vi "Charact Result Collection.vi"(0 "Operation":T1, 5 "Index":i32=1, 7 "Path cal resut In":variant) -> (4 "Path cal result out":variant, 6 "All path cal results":variant[](array[variant]))   [LabVIEW 2023, in "RFFixtureCharact.Public.lvlib"]
uses:
  RFFixtureCharact.Public.lvlib
  Type Definitions/Collection Operation.ctl
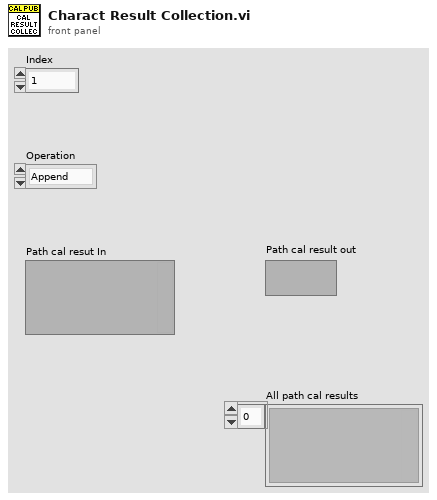
[diagram p1: front panel]
types:
  T1 = typedef "RFFixtureCharact.Public.lvlib/Collection Operation.ctl" = enum16{"Append", "Get", "Get All", "Clear"}
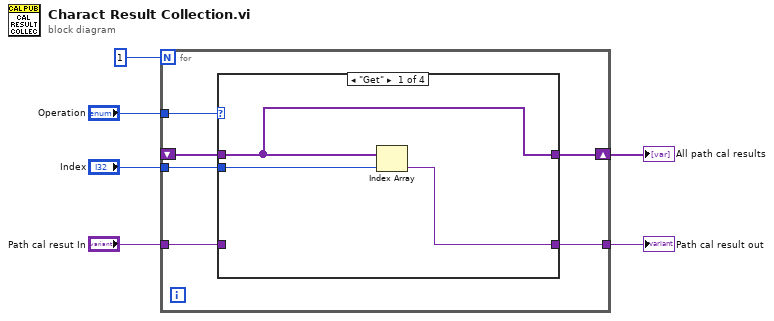
[diagram p0: block diagram]
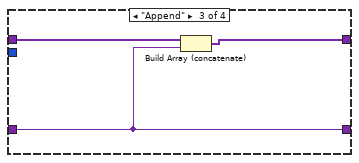
[diagram p3: hidden frame]
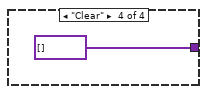
[diagram p4: hidden frame]
diagram:
  n1 = for {
    N: 1 -> [_]
    tunnel: [w12] -> w5
    shift-right: [w9] -> w1
    shift-left: _ -> [w10]
    tunnel: "Path cal resut In" -> [w11]
    tunnel: "Index" -> [w8]
    tunnel: "Operation" -> [w7]
    n2 = case shown="\"Get\"" w7 {
      tunnel: w10 -> [w15 w16 w19 _]
      tunnel: [w13 _ w18 _] -> w12
      tunnel: [w15 w16 w17 variant[] []] -> w9
      tunnel: w11 -> [_ _ w18 _]
      tunnel: w8 -> [w14 _ _ _]
      frame "Get" {
        n3 = Index Array(array=w15, index=w14) -> (element=w13:variant)
      }
      frame "Get All" {
      }
      frame "Append" {
        n4 = Build Array (concatenate)(w19, w18) -> (w17:variant[])
      }
      frame "Clear" {
      }
    }
  }
  "Path cal result out" <- w5
  "All path cal results" <- w1
